vi "CheckBeginScore.vi"(0 "object in":refnum<class "Play_v2.lvclass">, 3 "GameRef":refnum<data-value>, 5 "error in (no error)":errorcluster) -> (14 "object out":refnum<class "Play_v2.lvclass">, 16 "score":dbl, 19 "error out":errorcluster)   [LabVIEW 2023, in "Play_v2.lvclass"]
uses:
  Play_v2.lvclass
  Game_class/Game.lvclass
  Play_v2.lvclass/Play_v2.ctl
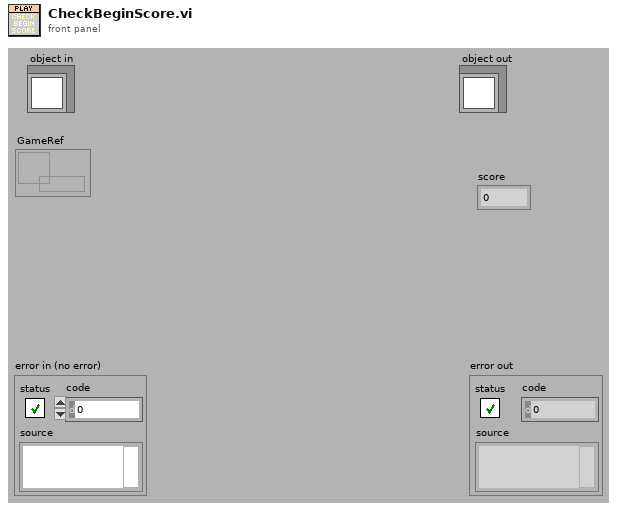
[diagram p1: front panel]
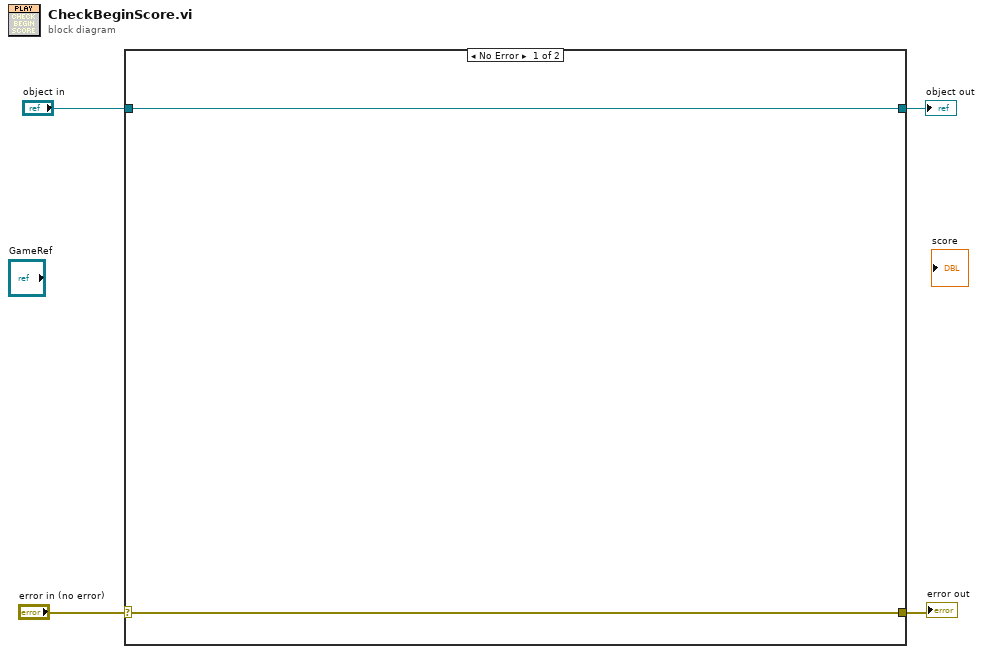
[diagram p0: block diagram]
diagram:
  n1 = case shown="No Error" "error in (no error)" {
    selector: "error in (no error)" -> [w6 w8]
    tunnel: [w6 w8] -> w3
    tunnel: [w5 w7] -> w1
    tunnel: "object in" -> [w5 w7]
    frame No Error {
    }
    frame Error {
    }
  }
  "error out" <- w3
  "object out" <- w1
